vi "Example SystemLink Alarm KPI Dashboard.vi"() -> ()   [LabVIEW 2019]
uses:
  <vilib>/Skyline/Alarm/Library/typedefs/Severity Level.ctl
  <vilib>/Skyline/Alarm/Filter Class/NI SystemLink Alarm Filter.lvclass
  <vilib>/Skyline/Alarm/Filter Class/NI SystemLink Alarm Filter.lvclass/NI SystemLink Alarm Filter.ctl
  <vilib>/Skyline/Configuration/Configuration HTTP_class/NI Skyline Configuration HTTP.lvclass/NI Skyline Configuration HTTP.ctl
  <vilib>/Skyline/Alarm/Class/NI SystemLink Alarm.lvclass/NI SystemLink Alarm.ctl
  <vilib>/Skyline/Configuration/Configuration HTTP_class/Open Configuration HTTP.vi
  <vilib>/Skyline/Alarm/Filter Class/Write Occurred After.vi
  <vilib>/Skyline/Alarm/Filter Class/Write Occurred Before.vi
  <vilib>/Skyline/Alarm/Filter Class/Read Filter.vi
  <vilib>/Skyline/Configuration/Configuration HTTP_class/Read Configuration.vi
  <vilib>/Skyline/Alarm/Filter Class/Write Highest Severity Level Min.vi
  <vilib>/Skyline/Alarm/Filter Class/Write Highest Severity Level Max.vi
  <vilib>/Skyline/Configuration/HTTP/Open Configuration (Desktop).vi
  <vilib>/Skyline/Alarm/Library/Query Alarms (With Transitions).vi
  <vilib>/Skyline/Alarm/Library/Query Alarms (No Transitions).vi
  <vilib>/Skyline/Configuration/Configuration HTTP_class/NI Skyline Configuration HTTP.lvclass
  <vilib>/Skyline/Alarm/Class/NI SystemLink Alarm.lvclass
  Library/SystemLink Alarm KPIs.lvlib
  <vilib>/Skyline/Alarm/Library/NI SystemLink Alarm Library.lvlib
  <vilib>/Skyline/Configuration/Configuration_class/NI Skyline Configuration.lvclass
panel:
  in  "Tab Control":T1(tab)
  out "Mean-Time-To-Resolution (days)":dbl format="%#.2g"
  out "Mean-Time-To-Ack (days)":dbl format="%#.2g"
  out "# of resolved (inactive) critical alarms":i32
  out "# of acknowledged critical alarms":i32
  out "Mean duration of alarms (days)":dbl format="%#.2g"
  out "# of active critical alarms":i32
  out "Mean-Time-To-Resolution (days)":dbl format="%#.2g"
  out "Mean-Time-To-Ack (days)":dbl format="%#.2g"
  out "# of resolved (inactive) non-critical alarms":i32
  out "# of acknowledged non-critical alarms":i32
  out "# of active non-critical alarms":i32
  out "Mean duration of alarms (days)":dbl format="%#.2g"
  out "# of Non-critical Alarms":i32
  out "# of Critical Alarms":i32
  in  "Occurred at or Before":timestamp
  in  "Occurred at or After":timestamp=timestamp(3692325600 s since 1904-01-01)
  # "Time Range of Alarms to Query"
  # "Lab Manager questions to answer:\n1. What needs to be fixed right now?  (how many active critical alarms)\n2. Am able to prevent critical incidents? (# of critical vs non-critical alarms)\n3. How fast is my staff able to respond to incidents? (MTTA)\n4. How fast is my staff able to fix/resolve incidents? (MTTR)\n\n5. How are these incident management metrics trending? (trend by month)"
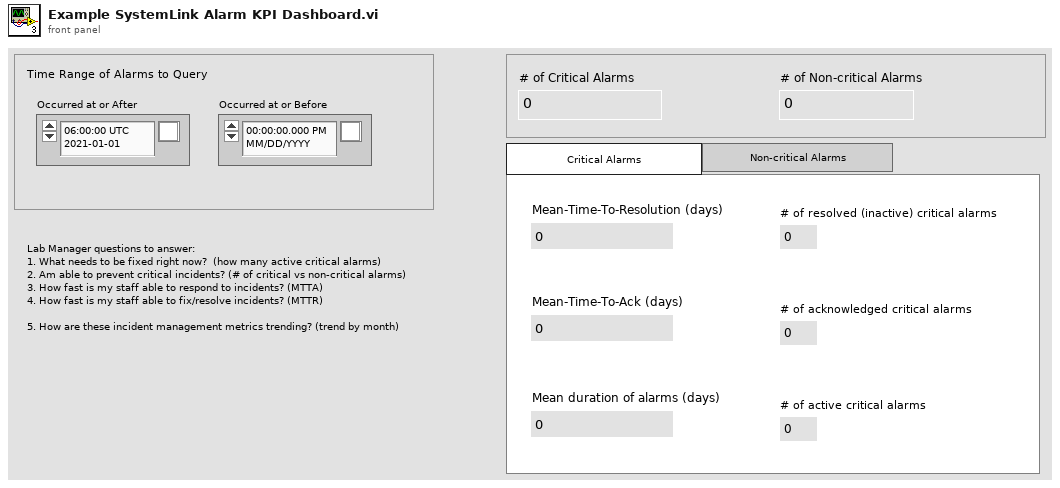
[diagram p1: front panel]
types:
  T1 = enum32{"Critical Alarms                                    ", "Non-critical Alarms                           "}
  T2 = typedef "NI SystemLink Alarm Library.lvlib/Severity Level.ctl" = i32
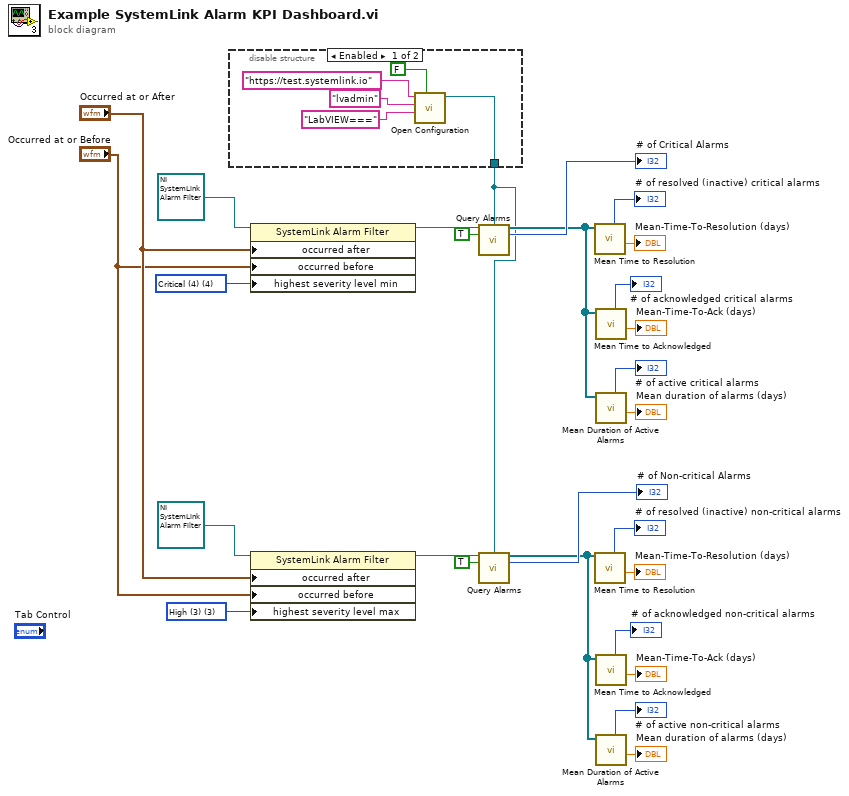
[diagram p0: block diagram]
diagram:
  w21 = T2 3 items=["Clear (-1)"=-1, "Low (1)"=1, "Moderate (2)"=2, "High (3)"=3, "Critical (4)"=4] ("highest severity level min")
  w25 = T2 4 items=["Clear (-1)"=-1, "Low (1)"=1, "Moderate (2)"=2, "High (3)"=3, "Critical (4)"=4] ("highest severity level min")
  n1 = disable-structure shown="Enabled" {
    disable-tunnel: [w29 _] -> w1
    frame Enabled {
      n2 = call-poly <vilib>:"Open Configuration.vi"("verify server?"=FALSE, "password"="LabVIEW===", "username"="lvadmin", "server url"="https://test.systemlink.io") -> ("configuration"=w29:refnum<class "NI Skyline Configuration HTTP.lvclass">)  [unwired: 6 in, 1 out]
    }
    frame Disabled {
    }
  }
  n3 = property class="SystemLink Alarm Filter"(reference=refnum<class "NI SystemLink Alarm Filter.lvclass"> refnum ("SystemLink Alarm Filter"), "occurred after"="Occurred at or After", "occurred before"="Occurred at or Before", "highest severity level min"=w25) -> (reference out=w26:refnum<class "NI SystemLink Alarm Filter.lvclass">)  [unwired: 1 in, 1 out]
  n4 = property class="SystemLink Alarm Filter"(reference=refnum<class "NI SystemLink Alarm Filter.lvclass"> refnum ("SystemLink Alarm Filter"), "occurred after"="Occurred at or After", "occurred before"="Occurred at or Before", "highest severity level max"=w21) -> (reference out=w20:refnum<class "NI SystemLink Alarm Filter.lvclass">)  [unwired: 1 in, 1 out]
  n5 = call <vilib>:"Query Alarms.vi"("filter"=w26, "HTTP configuration"=w1, "retrieve transitions?"=TRUE) -> ("alarms"=w2:refnum<class "NI SystemLink Alarm.lvclass">[], "total count"=→"# of Critical Alarms":i32)  [unwired: 10 in, 1 out]
  n6 = call <vilib>:"Query Alarms.vi"("filter"=w20, "HTTP configuration"=w1, "retrieve transitions?"=TRUE) -> ("alarms"=w7:refnum<class "NI SystemLink Alarm.lvclass">[], "total count"=→"# of Non-critical Alarms":i32)  [unwired: 10 in, 1 out]
  n7 = call "Mean Time to Resolution.vi"("alarms in"=w2) -> ("MTTR of inactive alarms (days)"=→"Mean-Time-To-Resolution (days)":dbl, "# of resolved (inactive) alarms"=→"# of resolved (inactive) critical alarms":i32)  [unwired: 5 in, 4 out]
  n8 = call "Mean Time to Resolution.vi"("alarms in"=w7) -> ("MTTR of inactive alarms (days)"=→"Mean-Time-To-Resolution (days)":dbl, "# of resolved (inactive) alarms"=→"# of resolved (inactive) non-critical alarms":i32)  [unwired: 5 in, 4 out]
  n9 = call "Mean Time to Acknowledged.vi"("alarms in"=w2) -> ("MTTA of alarms (days)"=→"Mean-Time-To-Ack (days)":dbl, "# of acknowledged alarms"=→"# of acknowledged critical alarms":i32)  [unwired: 5 in, 4 out]
  n10 = call "Mean Duration of Active Alarms.vi"("alarms in"=w2) -> ("Average duration of active alarms (days)"=→"Mean duration of alarms (days)":dbl, "#of active alarms"=→"# of active critical alarms":i32)  [unwired: 5 in, 4 out]
  n11 = call "Mean Time to Acknowledged.vi"("alarms in"=w7) -> ("MTTA of alarms (days)"=→"Mean-Time-To-Ack (days)":dbl, "# of acknowledged alarms"=→"# of acknowledged non-critical alarms":i32)  [unwired: 5 in, 4 out]
  n12 = call "Mean Duration of Active Alarms.vi"("alarms in"=w7) -> ("Average duration of active alarms (days)"=→"Mean duration of alarms (days)":dbl, "#of active alarms"=→"# of active non-critical alarms":i32)  [unwired: 5 in, 4 out]
